vi "SRV_InitVar.vi"(2 "Variable":T1) -> (0 "String":string)   [LabVIEW 2009]
panel:
  # "This LabVIEW item is deprecated.\n\nIt is believed to be unused and will be removed in a future version of SRV."
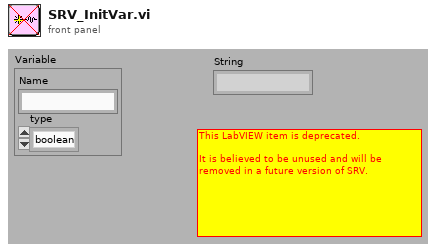
[diagram p1: front panel]
types:
  T1 = cluster{"Name":string, "type":enum16{"boolean", "u8", "i8", "u16", "i16", "u32", "i32", "u64", "i64", "SGL", "DBL", "EXT", "CPX"}}
  T2 = enum16{"boolean", "u8", "i8", "u16", "i16", "u32", "i32", "u64", "i64", "SGL", "DBL", "EXT", "CPX"}
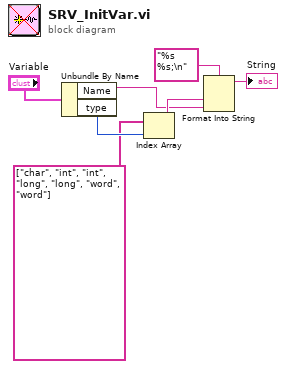
[diagram p0: block diagram]
diagram:
  n1 = Unbundle By Name("Variable") -> ("Name"=w5:string, "type"=w3:T2)
  n2 = Index Array(array=string[] ["char", "int", "int", "long", "long", "word", "word"], index=w3) -> (element=w6:string)
  n3 = Format Into String(format string="%s %s;\n", w6, w5) -> (resulting string=→"String":string)  [unwired: 2 in, 1 out]
